vi "BuildTeamSQLStrings.vi"(11 "BattleLog":T1) -> (3 "Team SQL INSERT request":string)   [LabVIEW 2020, in "StashRoyale.lvclass"]
uses:
  StashRoyale.lvclass
  ctl_BattleLog.ctl
  ctl_Team.ctl
  ctl_CardTeam.ctl
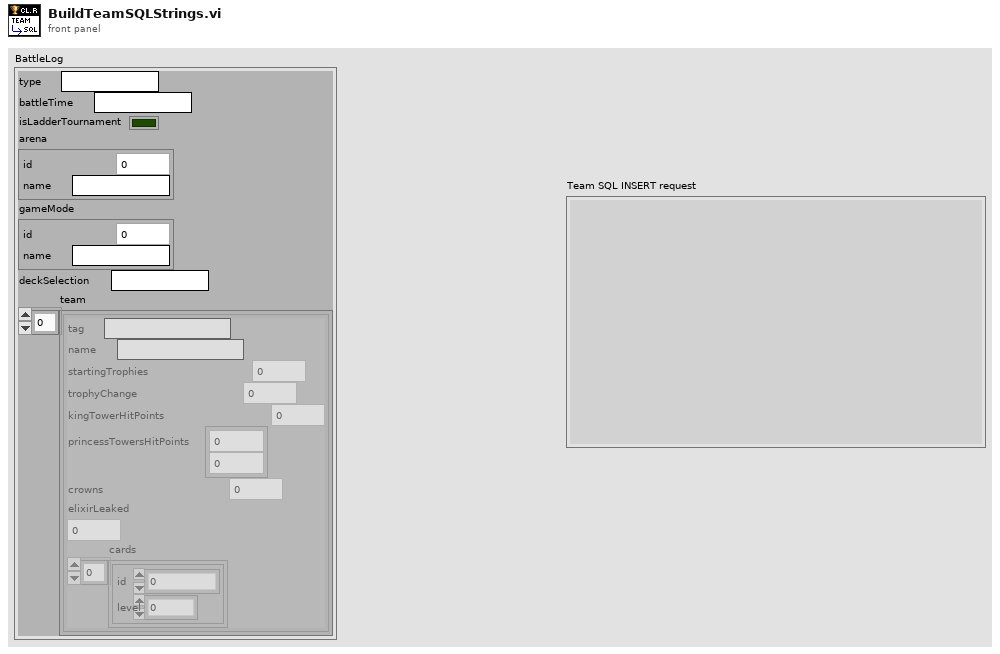
[diagram p1: front panel]
types:
  T1 = typedef "StashRoyale.lvclass/ctl_BattleLog.ctl" = cluster{"type":string, "battleTime":string, "isLadderTournament":bool, "arena":cluster{"id":u32, "name":string}, "gameMode":cluster{"id":u32, "name":string}, "deckSelection":string, "team":T2[]}
  T2 = typedef "ctl_Team.ctl" = cluster{"tag":string, "name":string, "startingTrophies":u16, "trophyChange":i16, "kingTowerHitPoints":u16, "princessTowersHitPoints":u16[], "crowns":u16, "elixirLeaked":sgl, "cards":T3[]}
  T3 = typedef "StashRoyale.lvclass/ctl_CardTeam.ctl" = cluster{"id":u32, "level":u8}
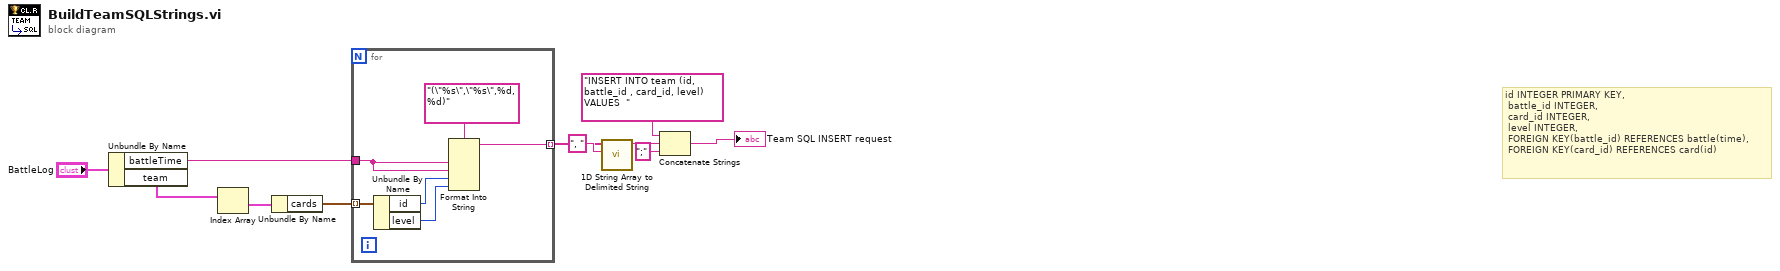
[diagram p0: block diagram]
diagram:
  # "id INTEGER PRIMARY KEY,\n\tbattle_id INTEGER,\n\tcard_id INTEGER,\n\tlevel INTEGER,\n\tFOREIGN KEY(battle_id) REFERENCES battle(time),\n\tFOREIGN KEY(card_id) REFERENCES card(id)"
  n1 = Unbundle By Name("BattleLog") -> ("battleTime"=w8:string, "team"=w10:T2[])
  n2 = Index Array(array=w10) -> (element=w9:T2)  [unwired: 1 in]
  n3 = Unbundle By Name(w9) -> ("cards"=w7:T3[])
  n4 = for {
    tunnel: w8 -> [w16]
    tunnel: w7 -> [w15] mode=indexing
    tunnel: [w12] -> w5 mode=indexing
    n5 = Unbundle By Name(w15) -> ("id"=w14:u32, "level"=w13:u8)
    n6 = Format Into String(format string="(\"%s\",\"%s\",%d, %d)", w16, w16, w14, w13) -> (resulting string=w12:string)  [unwired: 2 in, 1 out]
  }
  n7 = call <vilib>:"1D String Array to Delimited String.vi"("delimiter"=", ", "string array"=w5) -> ("delimited string"=w4:string)  [unwired: 9 in]
  n8 = Concatenate Strings("INSERT INTO team (id, battle_id , card_id, level) VALUES  ", w4, ";" ("string")) -> (→"Team SQL INSERT request":string)
